vi "Blink Stone Result.vi"(11 "String":u64) -> (2 "Single Digits":bool, 3 "Result Array":u64[](array[numeric]))   [LabVIEW 2024]
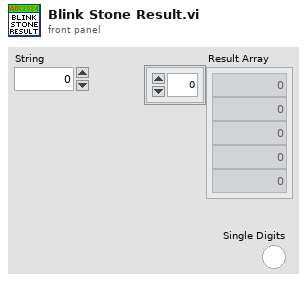
[diagram p1: front panel]
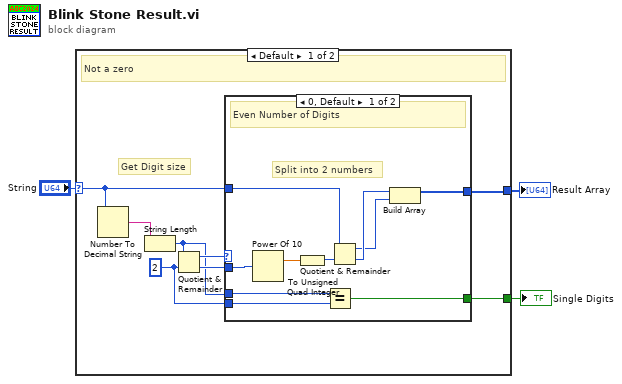
[diagram p0: block diagram]
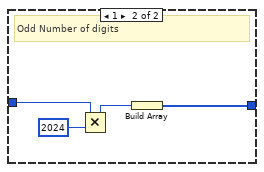
[diagram p2: hidden frame]
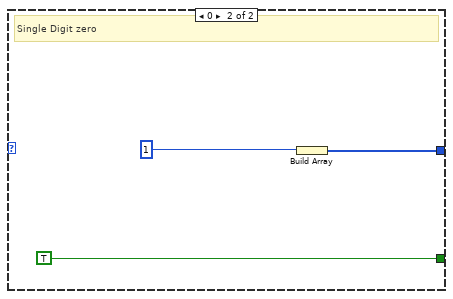
[diagram p3: hidden frame]
diagram:
  n1 = case shown="Default" "String" {
    selector: "String" -> [w10 _]
    tunnel: [w7 w27] -> w3
    tunnel: [w4 TRUE] -> w1
    frame Default {
      w6 = 2 ("y")
      # "Get Digit size"
      # "Not a zero"
      n2 = Number To Decimal String(number=w10) -> (decimal integer string=w8:string)  [unwired: 1 in]
      n3 = String Length(string=w8) -> (length=w5:i32)
      n4 = Quotient & Remainder(x=w5, y=w6) -> (x-y*floor(x/y)=w11:i32, floor(x/y)=w9:i32)
      n5 = case shown="0, Default" w11 {
        tunnel: w10 -> [w19 w25]
        tunnel: w9 -> [w21 _]
        tunnel: [w15 w22] -> w7
        tunnel: w6 -> [w14 _]
        tunnel: w5 -> [w13 _]
        tunnel: [w12 _] -> w4
        frame 0, Default {
          # "Split into 2 numbers"
          # "Even Number of Digits"
          n6 = Power Of 10(x=w21) -> (10^x=w20:dbl)
          n7 = To Unsigned Quad Integer(1:w20) -> (0:w18:u64)
          n8 = Equal?(x=w13, y=w14) -> (x = y?=w12:bool)
          n9 = Quotient & Remainder(x=w19, y=w18) -> (x-y*floor(x/y)=w16:u64, floor(x/y)=w17:u64)
          n10 = Build Array(w17, w16) -> (w15:u64[])
        }
        frame 1 {
          # "Odd Number of digits"
          n11 = Multiply(x=w25, y=u64 2024) -> (x*y=w23:u64)
          n12 = Build Array(w23) -> (w22:u64[])
        }
      }
    }
    frame 0 {
      # "Single Digit zero"
      n13 = Build Array(u64 1 ("String")) -> (w27:u64[])
    }
  }
  "Result Array" <- w3
  "Single Digits" <- w1
